vi "Example Simple.vi"() -> ()   [LabVIEW 2010]
uses:
  C:/tf/play/labview/Tinkerforge.dll
  Tinkerforge.dll
panel:
  out "w":sgl
  out "z":sgl
  out "y":sgl
  out "x":sgl
  in  "uid":string="6JpHZL"
  in  "port":i32=4223
  in  "host":string="localhost"
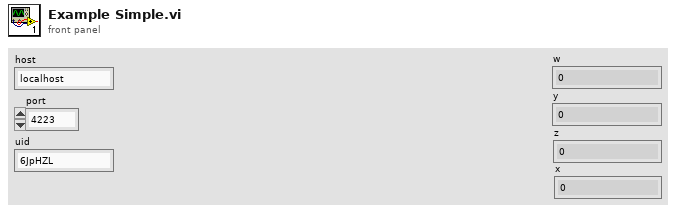
[diagram p1: front panel]
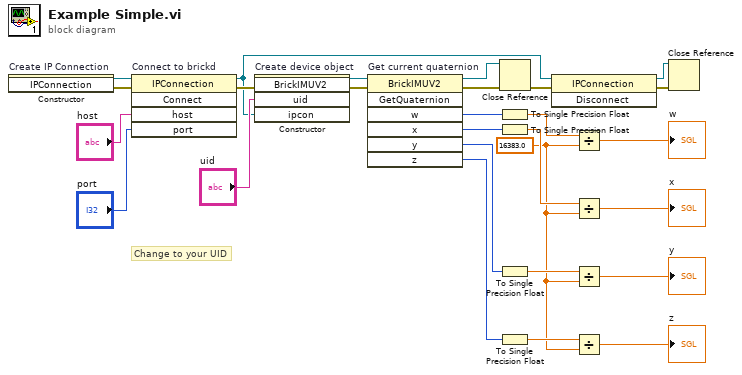
[diagram p0: block diagram]
diagram:
  w1 = sgl 16383.0 ("y")
  # "Change to your UID"
  n1 = constructor on="Create IP Connection" class="IPConnection"() -> (reference out=w27:refnum<k24>, error out=w14:errorcluster)  [unwired: 3 in, 1 out]
  n2 = invoke on="Connect to brickd" class="IPConnection" method="Connect"(reference=w27, error in=w14, "host"="host", "port"="port") -> (reference out=w16:refnum<k24>, error out=w23:errorcluster)  [unwired: 1 in, 3 out]
  n3 = constructor on="Create device object" class="BrickIMUV2"(error in=w23, "uid"="uid", "ipcon"=w16) -> (reference out=w21:refnum<k24>, error out=w22:errorcluster)  [unwired: 2 in, 3 out]
  n4 = invoke on="Get current quaternion" class="BrickIMUV2" method="GetQuaternion"(reference=w21, error in=w22) -> (reference out=w19:refnum<k24>, error out=w20:errorcluster, "w"=w11:i16, "x"=w4:i16, "y"=w3:i16, "z"=w2:i16)  [unwired: 5 in, 1 out]
  n5 = Close Reference(reference=w19, error in (no error)=w20) -> (error out=w18:errorcluster)
  n6 = To Single Precision Float(number=w11) -> (single precision float=w12:sgl)
  n7 = To Single Precision Float(number=w4) -> (single precision float=w10:sgl)
  n8 = To Single Precision Float(number=w3) -> (single precision float=w9:sgl)
  n9 = To Single Precision Float(number=w2) -> (single precision float=w8:sgl)
  n10 = invoke class="IPConnection" method="Disconnect"(reference=w16, error in=w18) -> (reference out=w15:refnum<k24>, error out=w17:errorcluster)  [unwired: 1 in, 1 out]
  n11 = Divide(x=w12, y=w1) -> (x/y=→"w":sgl)
  n12 = Divide(x=w10, y=w1) -> (x/y=→"x":sgl)
  n13 = Divide(x=w9, y=w1) -> (x/y=→"y":sgl)
  n14 = Divide(x=w8, y=w1) -> (x/y=→"z":sgl)
  n15 = Close Reference(reference=w15, error in (no error)=w17) -> ()  [unwired: 1 out]
